vi "receiveDataFromFPGA.vi"(8 "error in (no error)":errorcluster, 11 "ComponentData in":refnum<class "ComponentData.lvclass">) -> (0 "error out":errorcluster, 3 "ComponentData out":refnum<class "ComponentData.lvclass">)   [LabVIEW 2013, in "ComponentData.lvlib" / "ComponentData.lvclass"]
uses:
  <userlib>/Common/Component/common_application/RT/ComponentData/ComponentData/ComponentData.lvclass
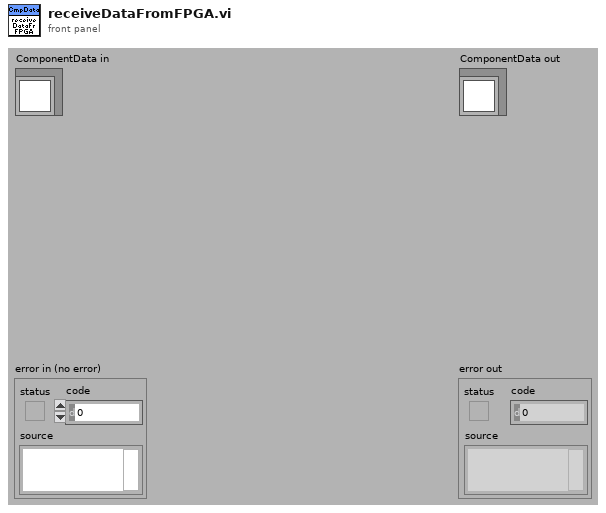
[diagram p1: front panel]
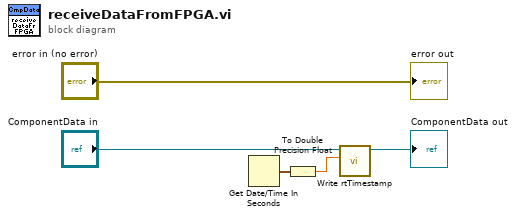
[diagram p0: block diagram]
diagram:
  n1 = Get Date/Time In Seconds() -> (seconds since 1Jan1904=w1:timestamp)
  n2 = To Double Precision Float(number=w1) -> (double precision float=w2:dbl)
  n3 = call <userlib>:"Write rtTimestamp.vi"("rtTimestamp"=w2, "ComponentData in"="ComponentData in") -> ("ComponentData out"=→"ComponentData out":refnum<class "ComponentData.lvclass">)  [unwired: 8 in, 1 out]
  "error out" <- "error in (no error)"
